vi "Plot Helper (Matrix).vi"(8 "error in (no error)":errorcluster, 9 "z matrix":sgl[][](array[numeric]), 10 "y vector":sgl[](array[numeric])) -> (0 "error out":errorcluster, 3 "3D Plot lvclass Array out":refnum<class "3D Plot Datatype.lvclass">[](array[class]))   [LabVIEW 2020, in "3D Bar Datatype.lvclass"]
doc: "Generates a plot of vertical bars."
uses:
  <vilib>/Math Plots/3D Math Plots/3D Bar/3D Bar Datatype/3D Bar Datatype.lvclass
  <vilib>/Math Plots/3D Math Plots/3D Plot/3D Plot Datatype/3D Plot Datatype.lvclass
  e:/builds/penguin/labview/branches/2020/dev/dist/vi.lib/Math Plots/3D Math Plots/3D Plot/3D Plot Datatype/3D Plot Datatype.lvclass
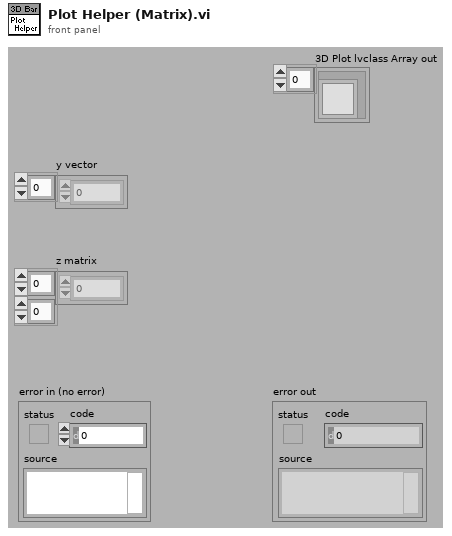
[diagram p1: front panel]
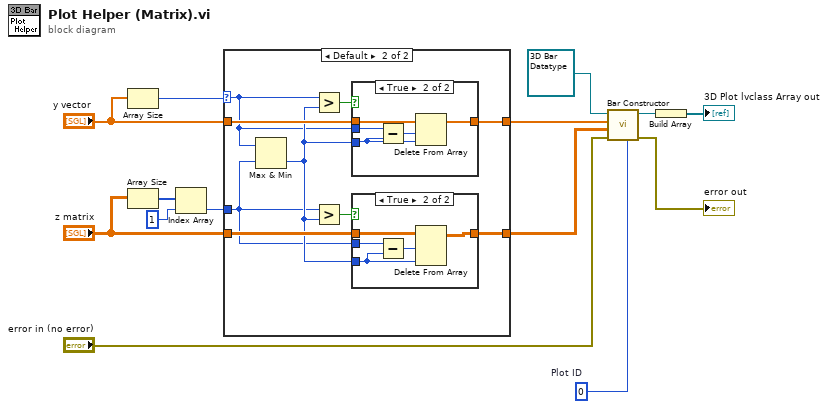
[diagram p0: block diagram]
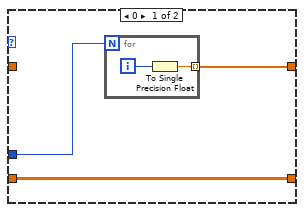
[diagram p2: hidden frame]
diagram:
  w9 = 0  # Plot ID
  n1 = Array Size(array="y vector") -> (size(s)=w1:i32)
  n2 = Array Size(array="z matrix") -> (size(s)=w4:i32[])
  n3 = Index Array(array=w4, index=1) -> (element=w2:i32)
  n4 = case shown="Default" w1 {
    selector: w1 -> [_ w21]
    tunnel: "y vector" -> [_ w28]
    tunnel: [w16 w27] -> w10
    tunnel: "z matrix" -> [w15 w26]
    tunnel: [w15 w25] -> w5
    tunnel: w2 -> [w17 w20]
    frame 0 {
      n5 = for {
        N: w17 -> [_]
        tunnel: [w18] -> w16 mode=indexing
        i -> [w19]
        n6 = To Single Precision Float(number=w19) -> (single precision float=w18:sgl)
      }
    }
    frame Default {
      n7 = Max & Min(x=w21, y=w20) -> (min(x,y)=w22:i32)  [unwired: 1 out]
      n8 = Greater?(x=w21, y=w22) -> (0:w23:bool)
      n9 = Greater?(x=w20, y=w22) -> (0:w24:bool)
      n10 = case shown="True" w23 {
        tunnel: w28 -> [w29 w34]
        tunnel: [w29 w33] -> w27
        tunnel: w22 -> [_ w31]
        tunnel: w21 -> [_ w32]
        frame False {
        }
        frame True {
          n11 = Subtract(x=w32, y=w31) -> (x-y=w30:i32)
          n12 = Delete From Array(array=w34, length=w30, index=w31) -> (array with subset deleted=w33:sgl[])  [unwired: 1 out]
        }
      }
      n13 = case shown="True" w24 {
        tunnel: w26 -> [w35 w40]
        tunnel: [w35 w39] -> w25
        tunnel: w22 -> [_ w37]
        tunnel: w20 -> [_ w38]
        frame False {
        }
        frame True {
          n14 = Subtract(x=w38, y=w37) -> (x-y=w36:i32)
          n15 = Delete From Array(array=w40, length=w36, index (col)=w37) -> (array with subset deleted=w39:sgl[][])  [unwired: 1 in, 1 out]
        }
      }
    }
  }
  n16 = call-dynamic "Bar Constructor.vi"("Plot ID"=w9, "error in (no error)"="error in (no error)", "z matrix"=w5, "y vector"=w10, "3D Bar Datatype.lvclass in"=refnum<class "3D Bar Datatype.lvclass"> refnum ("3D Mesh Datatype.lvclass")) -> ("error out"=→"error out":errorcluster, "3D Bar Datatype.lvclass out"=w8:refnum<class "3D Bar Datatype.lvclass">)  [unwired: 1 in, 4 out]
  n17 = Build Array(w8) -> (→"3D Plot lvclass Array out":refnum<class "3D Bar Datatype.lvclass">[])
